vi "SVPO Peak Level (N Ch DBL WDT).vi"(6 "restart averaging? (F)":bool, 11 "scaled signals [EU]":waveform(dbl)[](array[waveform])) -> (1 "minimum levels [EU]":dbl[](array[numeric]), 2 "maximum levels [EU]":dbl[](array[numeric]), 3 "peak levels [EU]":dbl[](array[numeric]), 4 "durations [s]":dbl[](array[numeric]), 5 "timestamps":timestamp[](array[timestamp]))   [LabVIEW 2017, in "SoundVib_VibrationLevel.lvlib"]
doc: "Uses a peak detector and computes the level of scaled time waveform signals and scaled array signals. <B>scaled signal [EU]</B> should have a zero DC component. You can attenuate the DC component with hardware AC-coupling filters and with software high-pass filters. Use this VI on embedded targets that have limited computational resources. Wire data to the scaled signal [EU] input to determine the polymorphic instance to use or manually select the instance."
uses:
  <vilib>/addons/Sound and Vibration/svt_Level/SoundVib_VibrationLevel.lvlib
  <vilib>/addons/_NISVFA/_Shared subVIs/Controls/svc_Peak Level State.ctl
  <vilib>/addons/Sound and Vibration/svt_Level/SVPO Peak Level (1 Ch DBL Array) with IC.vi
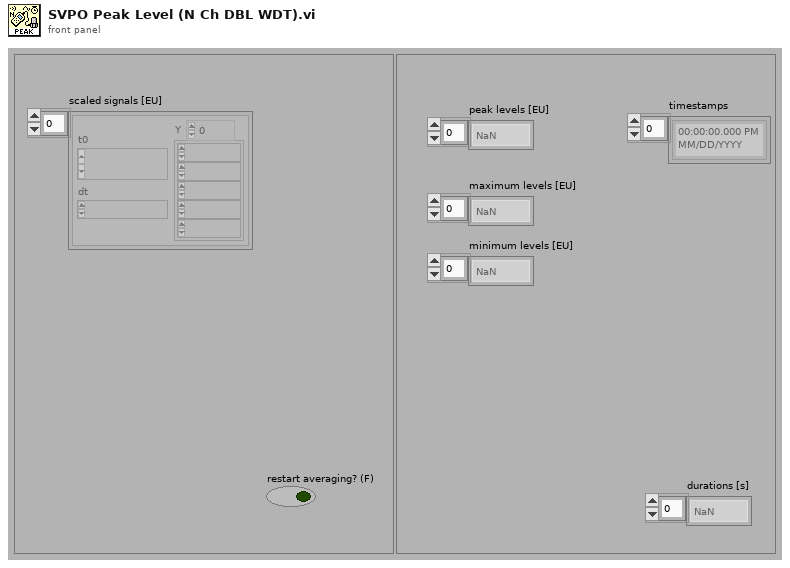
[diagram p1: front panel]
types:
  T1 = typedef "svc_Peak Level State.ctl" = cluster{"historical max":dbl, "historical min":dbl, "cumulative size":u64, "timestamp":timestamp}
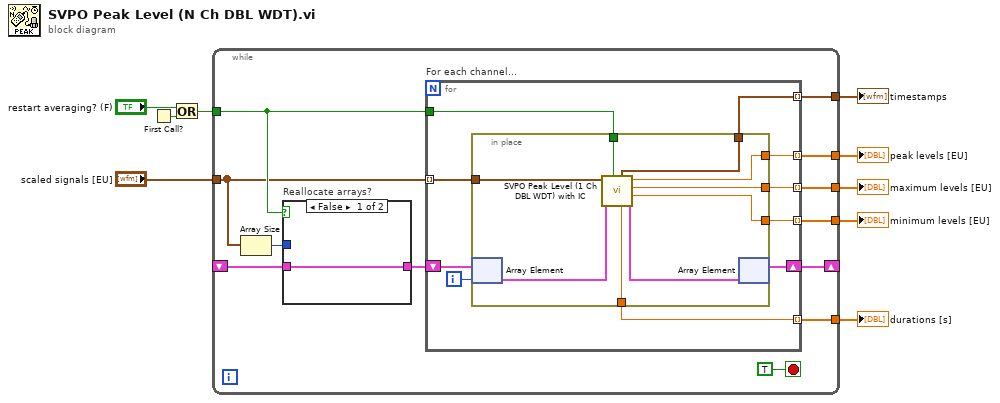
[diagram p0: block diagram]
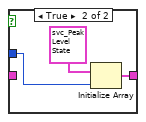
[diagram p2: hidden frame]
diagram:
  n1 = First Call?() -> (First Call?: T/F=w9:bool)
  n2 = Or(x="restart averaging? (F)", y=w9) -> (x .or. y?=w7:bool)
  n3 = while {
    tunnel: "scaled signals [EU]" -> [w11]
    tunnel: w7 -> [w16]
    shift-right: [w19] -> _
    shift-left: _ -> [w17]
    tunnel: [w18] -> w5
    tunnel: [w15] -> w4
    tunnel: [w14] -> w3
    tunnel: [w13] -> w2
    tunnel: [w12] -> w1
    stop <- TRUE stop-if-true
    n4 = Array Size(array=w11) -> (size(s)=w10:i32)
    n5 = case "Reallocate arrays?" shown="False" w16 {
      tunnel: [w22 w25] -> w20
      tunnel: w17 -> [w22 _]
      tunnel: w10 -> [_ w23]
      frame False {
      }
      frame True {
        n6 = Initialize Array(T1 {"historical max"=-inf, "historical min"=inf, "cumulative size"=0, "timestamp"=timestamp(0 s since 1904-01-01)} ("Initial Conditions"), w23) -> (w25:T1[])
      }
    }
    n7 = for "For each channel..." {
      tunnel: [w29] -> w18 mode=indexing
      tunnel: w16 -> [w35]
      tunnel: w11 -> [w30] mode=indexing
      shift-right: [w33] -> w19
      shift-left: w20 -> [w34]
      tunnel: [w31] -> w15 mode=indexing
      tunnel: [w28] -> w14 mode=indexing
      tunnel: [w27] -> w13 mode=indexing
      tunnel: [w26] -> w12 mode=indexing
      i -> [w32]
      n8 = in-place {
        in-place-border: w35 -> [w41]
        in-place-border: [w42] -> w31
        in-place-border: w30 -> [w40]
        in-place-border: [w39] -> w29
        in-place-border: [w38] -> w28
        in-place-border: [w37] -> w27
        in-place-border: [w36] -> w26
        n9 = in-place-array #1(w34, w32) -> (w44:T1)
        n10 = call <vilib>:"SVPO Peak Level (1 Ch DBL WDT) with IC.vi"("restart averaging? (F)"=w41, "initial conditions"=w44, "scaled signal [EU]"=w40) -> ("final conditions"=w43:T1, "minimum level [EU]"=w36:dbl, "maximum level [EU]"=w37:dbl, "peak level [EU]"=w38:dbl, "duration [s]"=w39:dbl, "timestamp"=w42:timestamp)  [unwired: 3 in]
        n11 = in-place-array #1(w43) -> (w33:T1[])  [unwired: 1 out]
      }
    }
  }
  "peak levels [EU]" <- w3
  "maximum levels [EU]" <- w2
  "minimum levels [EU]" <- w1
  "durations [s]" <- w5
  "timestamps" <- w4
